vi "bundle_4_AI_to_FIFO.vi"(5 "Input Valid":bool, 7 "FIFO In":refnum<k21>, 8 "AI3":i16, 9 "AI2":i16, 10 "AI1":i16, 11 "AI0":i16) -> (0 "Ready for Input":bool)   [LabVIEW 2015]
doc: "Bundles four Analog Input channel samples (U16) into a U64 FIFO. \nU64 is the largest built-in type.\nThis FIFO facilitates transfer between the 50MHz data aquisition loop and the 100MHz DRAM loop."
uses:
  <vilib>/rvi/DataTransferAndStorage/Container/Common/niFpgaContainerExecOnDevCompGetState.vi
  <vilib>/rvi/Emulation/niFpgaEmulationIsFPGAContextNoSignature.vi
  <vilib>/rvi/Emulation/niFpgaSctlEmulationGetInTimedLoop.vi
  <vilib>/rvi/errors/niFpgaSetErrorForExecOnDevCompSimple.vi
  <vilib>/rvi/eio/common/nirviEmuReportErrorAndStop.vi
  <vilib>/rvi/DataTransferAndStorage/Container/Common/niFpgaContainerGetUniqueNameForEmu.vi
  <vilib>/rvi/FIFO/Fifo_Resource/nirvififoEmulationSetSize.vi
  <vilib>/rvi/FIFO/Fifo_Resource/nirviFifoEmulationQueueMgr.vi
  <instcachedir>/0/nirviFifoEmulationQueueMgr_E5CAEC123FF24DC58D834DCA3CDAA9B5.lvgen/nirviFifoEmulationQueueMgr_E5CAEC123FF24DC58D834DCA3CDAA9B5_001.vi
  <vilib>/rvi/FIFO/Fifo_Resource/nirvififoEmulationDetermineInputValidOut.vi
  <vilib>/rvi/FIFO/Fifo_Resource/nirvififoEmulationCreateLock.vi
  <vilib>/rvi/Emulation/niFpgaProcessEmulError.vi
  <vilib>/rvi/FIFO/Fifo_Resource/nirvififoEmulationObtainLock.vi
  <vilib>/rvi/FIFO/Fifo_Resource/nirvififoEmulationReleaseLock.vi
  <vilib>/rvi/occurrence/nirviWaitOnOccurrenceBase.vi
  <vilib>/rvi/errors/nirviReportUnexpectedCaseInternalError.vi
  <vilib>/rvi/errors/nirviReportUnexpectedCaseInternalError (U32).vi
  <vilib>/Utility/error.llb/Clear Errors.vi
  <vilib>/rvi/interface/RandomDataEmulation/niFpgaRandomDataHandleErrors.vi
  <vilib>/rvi/DataTransferAndStorage/Container/XNode/niFpgaContainer.xnode
  <vilib>/rvi/FIFO/Fifo_Resource/niFpgaFifoEmulationRefIn.vi
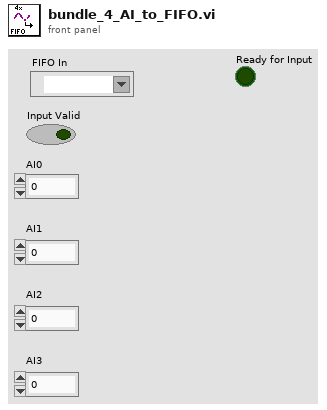
[diagram p1: front panel]
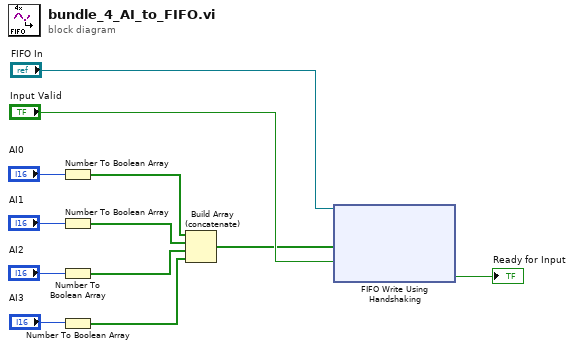
[diagram p0: block diagram]
diagram:
  n1 = Number To Boolean Array(number="AI0") -> (Boolean array=w8:bool[])
  n2 = Number To Boolean Array(number="AI1") -> (Boolean array=w7:bool[])
  n3 = Number To Boolean Array(number="AI2") -> (Boolean array=w4:bool[])
  n4 = Number To Boolean Array(number="AI3") -> (Boolean array=w5:bool[])
  n5 = Build Array (concatenate)(w8, w7, w4, w5) -> (w2:bool[])
  n6 = xnode ("FIFO Write Using Handshaking")("Element"=w2, "Input Valid"="Input Valid", "FIFO In"="FIFO In") -> ("Ready for Input"=→"Ready for Input":bool)  [unwired: 1 out]
